vi "Demo EV3-OnShape.vi"() -> ()   [LabVIEW 2019]
uses:
  <userlib>/Onshape/_SubVI/z did wid and eid.vi
  <userlib>/Onshape Feature Functions/_SubVI/FS Body Cuboid.vi
panel:
  in  "Enter your IP address":string="10.0.0.161"
  in  "Cuboid":T1={"Point 1"={"x"=0.0, "y"=0.0, "z"=0.0}, "Point 2"={"x"=1.0, "y"=1.0, "z"=1.0}}
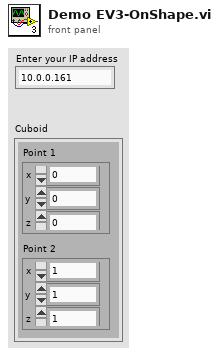
[diagram p1: front panel]
types:
  T1 = cluster{"Point 1":cluster{"x":dbl, "y":dbl, "z":dbl}, "Point 2":cluster{"x":dbl, "y":dbl, "z":dbl}}
  T2 = cluster{"y1":i32, "x1":i32, "x2":i32, "y2":i32, "extrude":i32, "setflag":string}
  T3 = typedef "Cluster.ctl" = cluster{"Date":string, "On-Nonce":string, "eid":string, "wid":string, "did":string, "name":string, "method":string, "Accept":string, "User-Agent":string, "Content-Type":string, "stack":string, "headers":string[], "payload":string, "ctype":string, "path":string, "Authorization":string, "secret_key":string, "access_key":string}
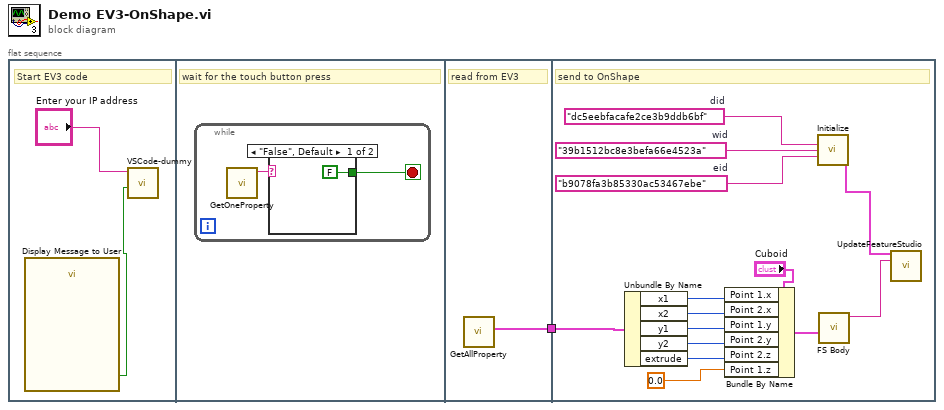
[diagram p0: block diagram]
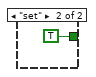
[diagram p2: hidden frame]
diagram:
  n1 = flat-sequence {
    tunnel: [w8] -> w1
    tunnel: w1 -> [w21]
    frame #0 {
      # "Start EV3 code"
      n2 = call "Display Message to User"() -> ("OK"=w2:bool)  [unwired: 10 in, 1 out]
      n3 = call <userlib>:"VSCode-dummy.vi"("Make new code?"=w2, "Enter your IP address"="Enter your IP address") -> ()  [unwired: 8 in, 2 out]
    }
    frame #1 {
      # "wait for the touch button press"
      n4 = while {
        stop <- w4 stop-if-true
        n5 = call <userlib>:"GetOneProperty.vi"() -> ("setflag"=w5:string)  [unwired: 10 in, 1 out]
        n6 = case shown="\"False\", Default" w5 {
          tunnel: [FALSE TRUE] -> w4
          frame "False", Default {
          }
          frame "set" {
          }
        }
      }
    }
    frame #2 {
      # "read from EV3"
      n7 = call <userlib>:"GetAllProperty.vi"() -> ("element"=w8:T2)  [unwired: 10 in, 1 out]
    }
    frame #3 {
      w9 = "b9078fa3b85330ac53467ebe"  # eid
      w10 = "39b1512bc8e3befa66e4523a"  # wid
      w11 = "dc5eebfacafe2ce3b9ddb6bf"  # did
      # "send to OnShape"
      n8 = Unbundle By Name(w21) -> ("x1"=w19:i32, "x2"=w18:i32, "y1"=w17:i32, "y2"=w16:i32, "extrude"=w15:i32)
      n9 = Bundle By Name(cluster="Cuboid", "Point 1.x"=w19, "Point 2.x"=w18, "Point 1.y"=w17, "Point 2.y"=w16, "Point 2.z"=w15, "Point 1.z"=0.0) -> (w13:T1)
      n10 = call-poly <userlib>:"Initialize.vi"("did"=w11, "wid"=w10, "eid"=w9) -> ("Device Out"=w22:T3)  [unwired: 11 in, 1 out]
      n11 = call-poly <userlib>:"FS Body.vi"("Cuboid"=w13) -> ("Feature Out"=w12:string)  [unwired: 10 in]
      n12 = call <userlib>:"UpdateFeatureStudio.vi"("Device In"=w22, "FeatureScript"=w12) -> ()  [unwired: 11 in, 3 out]
    }
  }
